vi "check for accepted connections.vi"(8 "error in":errorcluster, 9 "timeout":i32=1000, 11 "server acceptor in":refnum<class "server acceptor.lvclass">) -> (0 "error out":errorcluster, 3 "connection":refnum<class "connection.lvclass">)   [LabVIEW 2016, in "server acceptor.lvclass"]
uses:
  server acceptor.lvclass
  connection/connection.lvclass
  server acceptor.lvclass/server acceptor.ctl
  dllwrapper/async tls dl.lvlib
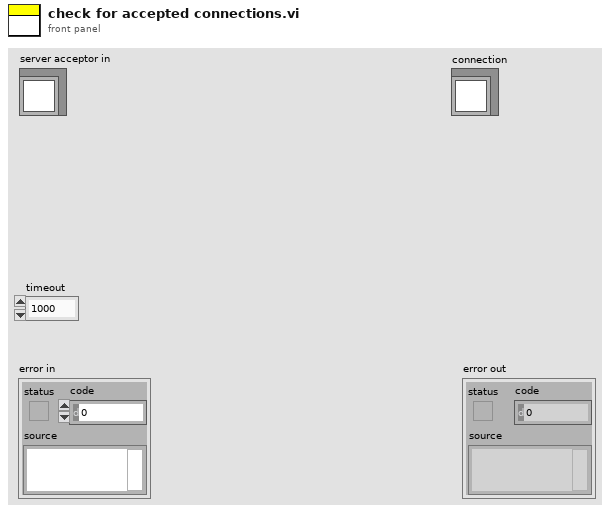
[diagram p1: front panel]
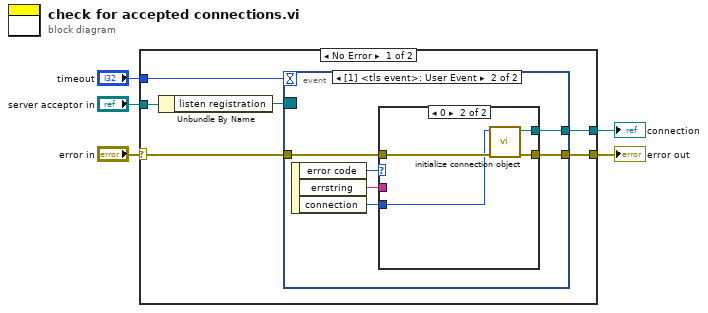
[diagram p0: block diagram]
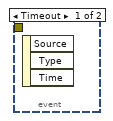
[diagram p2: hidden frame]
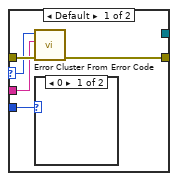
[diagram p3: hidden frame]
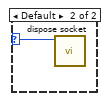
[diagram p4: hidden frame]
diagram:
  n1 = case shown="No Error" "error in" {
    selector: "error in" -> [w8 w28]
    tunnel: [w7 w28] -> w4
    tunnel: "server acceptor in" -> [w11 _]
    tunnel: "timeout" -> [w9 _]
    tunnel: [w6 _] -> w1
    frame No Error {
      n2 = Unbundle By Name(w11) -> ("listen registration"=w10:refnum<event-registration>)
      n3 = event shown="[1] <tls event>: User Event" {
        selector: w10 -> [_ _]
        dyn-events: _ -> [_ _]
        timeout: w9 -> [_ _]
        tunnel: w8 -> [_ w17]
        tunnel: [_ w14] -> w7
        tunnel: [_ w16] -> w6
        event Timeout {
          n4 = event-data() -> ()  [unwired: 1 in, 3 out]
        }
        event User Event {
          n5 = event-data() -> ("error code"=w13:i32, "errstring"=w12:string, "connection"=w15:u64)  [unwired: 1 in]
          n6 = case shown="0" w13 {
            selector: w13 -> [w19 _]
            tunnel: w17 -> [w22 w27]
            tunnel: [_ w26] -> w16
            tunnel: w15 -> [w18 w25]
            tunnel: [w21 w24] -> w14
            tunnel: w12 -> [w20 _]
            frame Default {
              n7 = call <vilib>:"Error Cluster From Error Code.vi"("error in (no error)"=w22, "error message (\"\")"=w20, "error code (0)"=w19) -> ("error out"=w21:errorcluster)  [unwired: 6 in]
              n8 = case shown="0" w18 {
                selector: w18 -> [_ w23]
                frame 0 {
                }
                frame Default {
                  n9 = call "dispose socket.vi"("socket"=w23) -> ()  [unwired: 10 in, 1 out]
                }
              }
            }
            frame 0 {
              n10 = call "initialize connection object.vi"("error in"=w27, "connection"=w25) -> ("error out"=w24:errorcluster, "connection out"=w26:refnum<class "connection.lvclass">)  [unwired: 8 in]
            }
          }
        }
      }
    }
    frame Error {
    }
  }
  "error out" <- w4
  "connection" <- w1
